vi "ListCollections.vi"(8 "error in (no error)":errorcluster, 11 "MongoDB-Database in":refnum<class "MongoDB-Database.lvclass">) -> (0 "error out":errorcluster, 2 "ListCollections":string[](array[string]), 3 "MongoDB-Database out":refnum<class "MongoDB-Database.lvclass">)   [LabVIEW 2016, in "MongoDB-Database.lvlib" / "MongoDB-Database.lvclass"]
uses:
  MongoDB-Database.lvclass
  D:/Users/blume/Desktop/LV/MongoDB-Driver/MLV DLLs/MongoLabVIEW.dll
  LV/MongoDB-Driver/MLV DLLs/MongoLabVIEW.dll
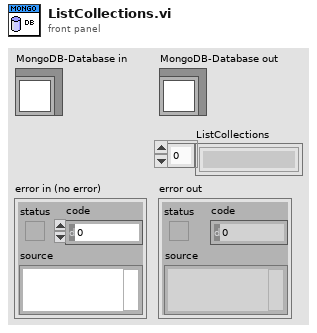
[diagram p1: front panel]
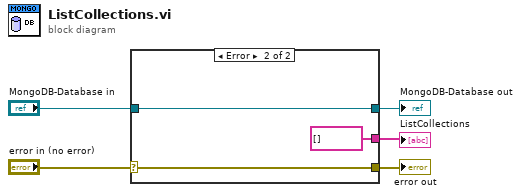
[diagram p0: block diagram]
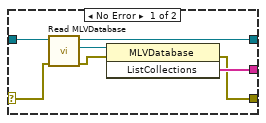
[diagram p2: hidden frame]
diagram:
  n1 = case shown="Error" "error in (no error)" {
    selector: "error in (no error)" -> [w11 w15]
    tunnel: [w6 w15] -> w4
    tunnel: [w8 w14] -> w2
    tunnel: "MongoDB-Database in" -> [w12 w14]
    tunnel: [w7 string[] [] ("ListCollections")] -> w1
    frame No Error {
      n2 = call "Read MLVDatabase.vi"("error in (no error)"=w11, "MongoDB-Database in"=w12) -> ("error out"=w9:errorcluster, "MLVDatabase"=w10:refnum<k24>, "MongoDB-Database out"=w8:refnum<class "MongoDB-Database.lvclass">)  [unwired: 7 in]
      n3 = invoke class="MLVDatabase" method="ListCollections"(reference=w10, error in=w9) -> (error out=w6:errorcluster, "ListCollections"=w7:string[])  [unwired: 1 in, 1 out]
    }
    frame Error {
    }
  }
  "error out" <- w4
  "MongoDB-Database out" <- w2
  "ListCollections" <- w1
